vi "SSL_load_error_strings.vi"(8 "error in (no error)":errorcluster, 11 "SSL-Lib in":refnum<class "SSL-Lib.lvclass">) -> (0 "error out":errorcluster, 3 "SSL-Lib out":refnum<class "SSL-Lib.lvclass">)   [LabVIEW 2013, in "SSL_Lib.lvlib" / "SSL-Lib.lvclass"]
uses:
  SSL-Lib.lvclass
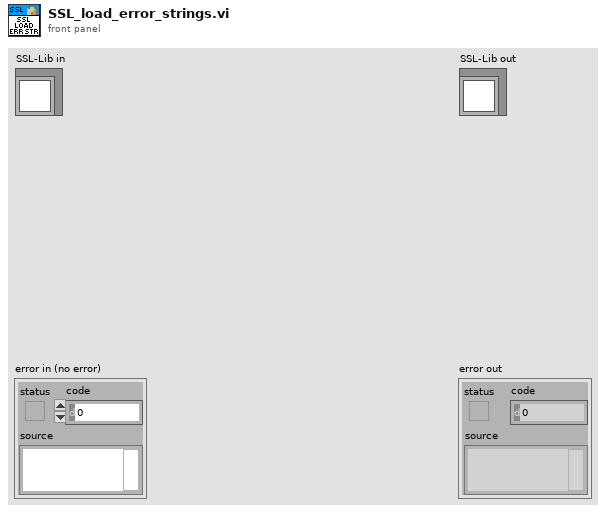
[diagram p1: front panel]
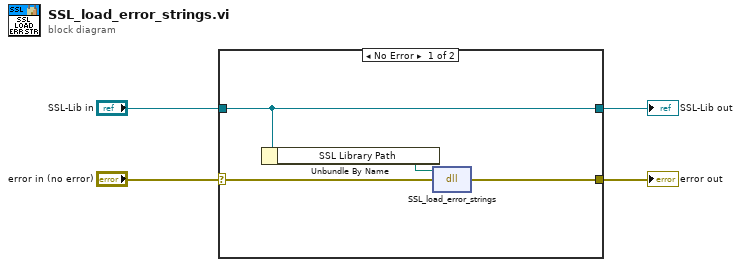
[diagram p0: block diagram]
diagram:
  n1 = case shown="No Error" "error in (no error)" {
    selector: "error in (no error)" -> [w8 w10]
    tunnel: [w5 w10] -> w3
    tunnel: [w7 w9] -> w1
    tunnel: "SSL-Lib in" -> [w7 w9]
    frame No Error {
      n2 = Unbundle By Name(w7) -> ("SSL Library Path"=w6:path)
      n3 = dll-call lib="C:/Program Files (x86)/National Instruments/Shared/nissl/NIssleay32.dll" fn="SSL_load_error_strings"(path in=w6, error in=w8) -> (error out=w5:errorcluster)  [unwired: 2 in, 1 out]
    }
    frame Error {
    }
  }
  "error out" <- w3
  "SSL-Lib out" <- w1
